vi "Retentive Timer On.vi"(8 "error in":errorcluster, 9 "reset":bool, 10 "preset time":i32=1000, 11 "enable":bool) -> (0 "error out":errorcluster, 2 "done":bool, 3 "accumulated time":i32)   [LabVIEW 2017, in "NI_FunctionBlock Libraries.lvlib"]
uses:
  <vilib>/functionblocks/NI_FunctionBlock Libraries.lvlib
  <vilib>/ptbypt/NI_PtbyPt.lvlib
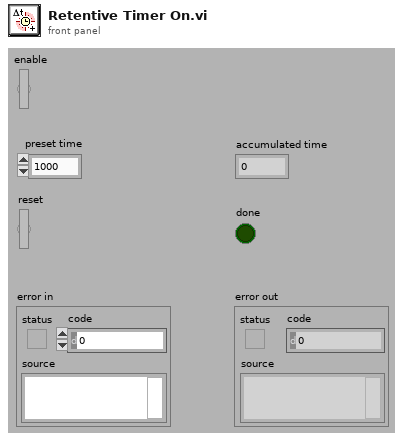
[diagram p1: front panel]
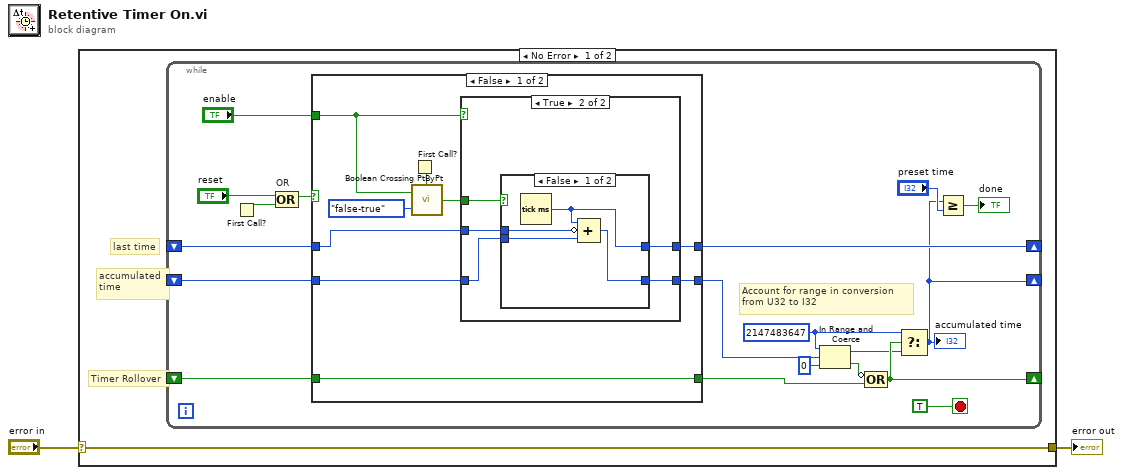
[diagram p0: block diagram]
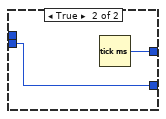
[diagram p3: hidden frame]
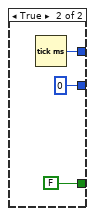
[diagram p4: hidden frame]
diagram:
  n1 = case shown="No Error" "error in" {
    selector: "error in" -> [w3 w48]
    tunnel: [w3 w48] -> w1
    frame No Error {
      # "Timer Rollover"
      # "accumulated\ntime"
      # "last time"
      n2 = while {
        shift-left: _ -> [w19]
        shift-right: [w20] -> _
        shift-right: [w4] -> _
        shift-left: _ -> [w16]
        shift-right: [w8] -> _
        shift-left: _ -> [w7]
        stop <- TRUE stop-if-true
        w10 = u32 2147483647 ("upper limit")
        # "Account for range in conversion\nfrom U32 to I32"
        n3 = First Call?() -> (First Call?: T/F=w17:bool)
        n4 = Compound Arithmetic op=OR "OR"("reset", w17) -> (w21:bool)
        n5 = case shown="False" w21 {
          tunnel: [w28 w47] -> w20
          tunnel: w19 -> [w31 _]
          tunnel: w16 -> [w30 _]
          tunnel: "enable" -> [w25 _]
          tunnel: [w29 0] -> w9
          tunnel: w7 -> [w23 _]
          tunnel: [w23 FALSE] -> w6
          frame False {
            n6 = First Call?() -> (First Call?: T/F=w26:bool)
            n7 = call <vilib>:"Boolean Crossing PtByPt.vi"("initialize"=w26, "direction"=enum16{"either", "false-true", "true-false"}."false-true", "input"=w25) -> ("crossing"=w24:bool)
            n8 = case shown="True" w25 {
              tunnel: w31 -> [w32 w38]
              tunnel: w30 -> [w33 w37]
              tunnel: [w33 w35] -> w29
              tunnel: [w32 w36] -> w28
              tunnel: w24 -> [_ w34]
              frame False {
              }
              frame True {
                n9 = case shown="False" w34 {
                  tunnel: w38 -> [w42 _]
                  tunnel: w37 -> [w41 w44]
                  tunnel: [w40 w43] -> w36
                  tunnel: [w39 w44] -> w35
                  frame False {
                    n10 = Tick Count (ms)() -> (millisecond timer value=w40:u32)
                    n11 = Compound Arithmetic op=ADD(w40, invert w42, w41) -> (w39:u32)
                  }
                  frame True {
                    n12 = Tick Count (ms)() -> (millisecond timer value=w43:u32)
                  }
                }
              }
            }
          }
          frame True {
            n13 = Tick Count (ms)() -> (millisecond timer value=w47:u32)
          }
        }
        n14 = In Range and Coerce(upper limit=w10, x=w9, lower limit=u32 0) -> (coerced(x)=w5:u32, In Range?=w11:bool)
        n15 = Compound Arithmetic op=OR(invert w11, w6) -> (w8:bool)
        n16 = Select(t=w10, s=w8, f=w5) -> (s? t:f=w4:u32)
        "accumulated time" <- w4
        n17 = Greater Or Equal?(x=w4, y="preset time") -> (x >= y?=→"done":bool)
      }
    }
    frame Error {
    }
  }
  "error out" <- w1
